vi "Send Set DER GenerationMode Msg (Delayed).vi"(7 "Milliseconds To Wait (1000)":i32=1000, 8 "error in":errorcluster, 10 "DER_setGenerationMode":T1, 11 "SCADA Sub Abstract in":refnum<class "Device Communication and Control Abstract.lvclass">) -> (0 "error out":errorcluster, 3 "dup SCADA Sub Abstract":refnum<class "Device Communication and Control Abstract.lvclass">)   [LabVIEW 2018, in "Device Communication and Control Abstract Actor.lvlib" / "Device Communication and Control Abstract.lvclass"]
uses:
  Device Communication and Control Abstract.lvclass
  C:/Program Files (x86)/National Instruments/LabVIEW 2018/vi.lib/ActorFramework/Actor/Actor.lvclass
  <vilib>/ORNL/CSEISMIC DDS/CSEISMIC DDS Base/Data Types/DER_setGenerationMode.ctl
  <vilib>/ORNL/CSEISMIC DDS/CSEISMIC DDS Base/Data Types/Controls/DeviceID.ctl
  <vilib>/ORNL/CSEISMIC DDS/CSEISMIC DDS Base/Data Types/Controls/Generation Mode.ctl
  <vilib>/ActorFramework/Actor/Actor.lvclass/Actor.ctl
  Device Communication and Control Abstract.lvclass/Device Communication and Control Abstract.ctl
  Device Communication and Control Abstract Messages/Set DER GenerationMode Msg/Set DER GenerationMode Msg.lvclass/Set DER GenerationMode Msg.ctl
  Device Communication and Control Abstract Messages/Set DER GenerationMode Msg/Set DER GenerationMode Msg.lvclass
  C:/Program Files (x86)/National Instruments/LabVIEW 2018/vi.lib/ActorFramework/Message/Message.lvclass
  <vilib>/ActorFramework/Time-Delayed Send Message/Time-Delayed Send Message.vi
  <vilib>/ActorFramework/Actor/Actor.lvclass
  <vilib>/ORNL/CSEISMIC DDS/CSEISMIC DDS Base/CSEISMIC DDS.lvclass
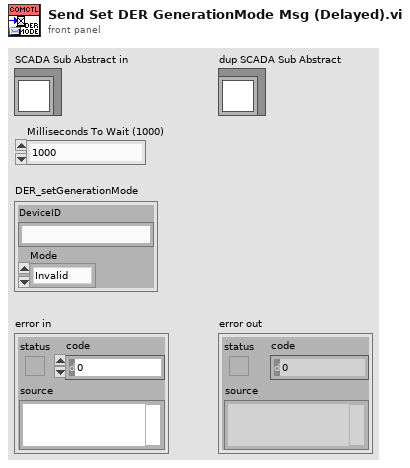
[diagram p1: front panel]
types:
  T1 = typedef "CSEISMIC DDS.lvlib/CSEISMIC DDS.lvclass/DER_setGenerationMode.ctl" = cluster{"DeviceID":T2, "Mode":T3}
  T2 = typedef "CSEISMIC DDS.lvlib/CSEISMIC DDS.lvclass/DeviceID.ctl" = string
  T3 = typedef "CSEISMIC DDS.lvlib/CSEISMIC DDS.lvclass/Generation Mode.ctl" = enum32{"Invalid", "PQ", "Droop", "PV", "PF", "VF"}
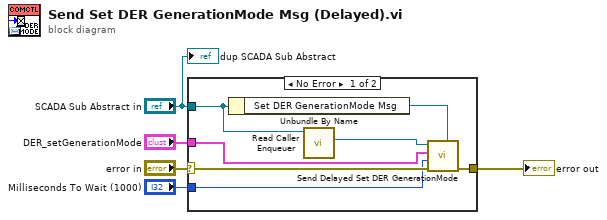
[diagram p0: block diagram]
diagram:
  n1 = case shown="No Error" "error in" {
    selector: "error in" -> [w9 w13]
    tunnel: "SCADA Sub Abstract in" -> [w12 _]
    tunnel: "DER_setGenerationMode" -> [w8 _]
    tunnel: [w7 w13] -> w2
    tunnel: "Milliseconds To Wait (1000)" -> [w6 _]
    frame No Error {
      n2 = Unbundle By Name(w12) -> ("Set DER GenerationMode Msg"=w10:refnum<class "Set DER GenerationMode Msg.lvclass">)
      n3 = call <vilib>:"Read Caller Enqueuer.vi"("Actor"=w12) -> ("Caller Enqueuer"=w11:refnum<class "Message Enqueuer.lvclass">)  [unwired: 10 in]
      n4 = call "Send Delayed Set DER GenerationMode.vi"("Message Type"=w10, "error in (no error)"=w9, "Milliseconds To Wait"=w6, "DER_setGenerationMode"=w8, "Message Enqueuer"=w11) -> ("error out"=w7:errorcluster)  [unwired: 5 in, 1 out]
    }
    frame Error {
    }
  }
  "error out" <- w2
  "dup SCADA Sub Abstract" <- "SCADA Sub Abstract in"
